vi "Parallel Loops - Pre izmene.vi"() -> ()   [LabVIEW 2016]
panel:
  out "Iter Akvizicija":i32
  out "Real":dbl
  out "Z":bool
  out "Y":bool
  out "X":bool
  in  "Treshold":dbl=1.0999999999999999 min=0.0 max=5.0 step=0.1
  out "Akvizicija":bool
  out "ACC1 Z":dbl
  out "ACC1 Y":dbl
  out "ACC1 X":dbl
  out "data":dynamicdata(graph)
  in  "Akvizicija - Error":string="N/A"
  out "Iter Sekvenca":i32
  in  "stop":bool
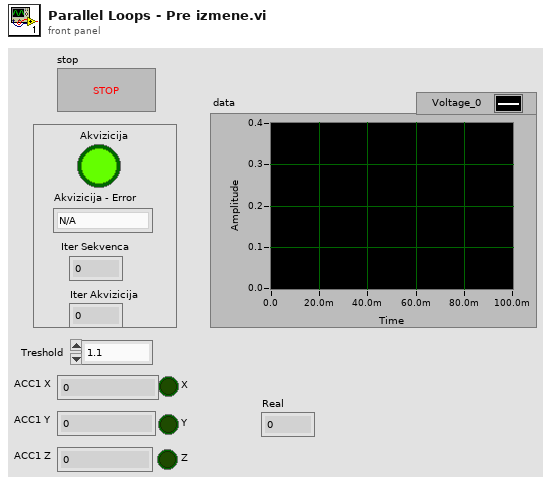
[diagram p1: front panel]
types:
  T1 = enum16{"open", "replace", "create", "open or create", "replace or create", "replace or create with confirmation"}
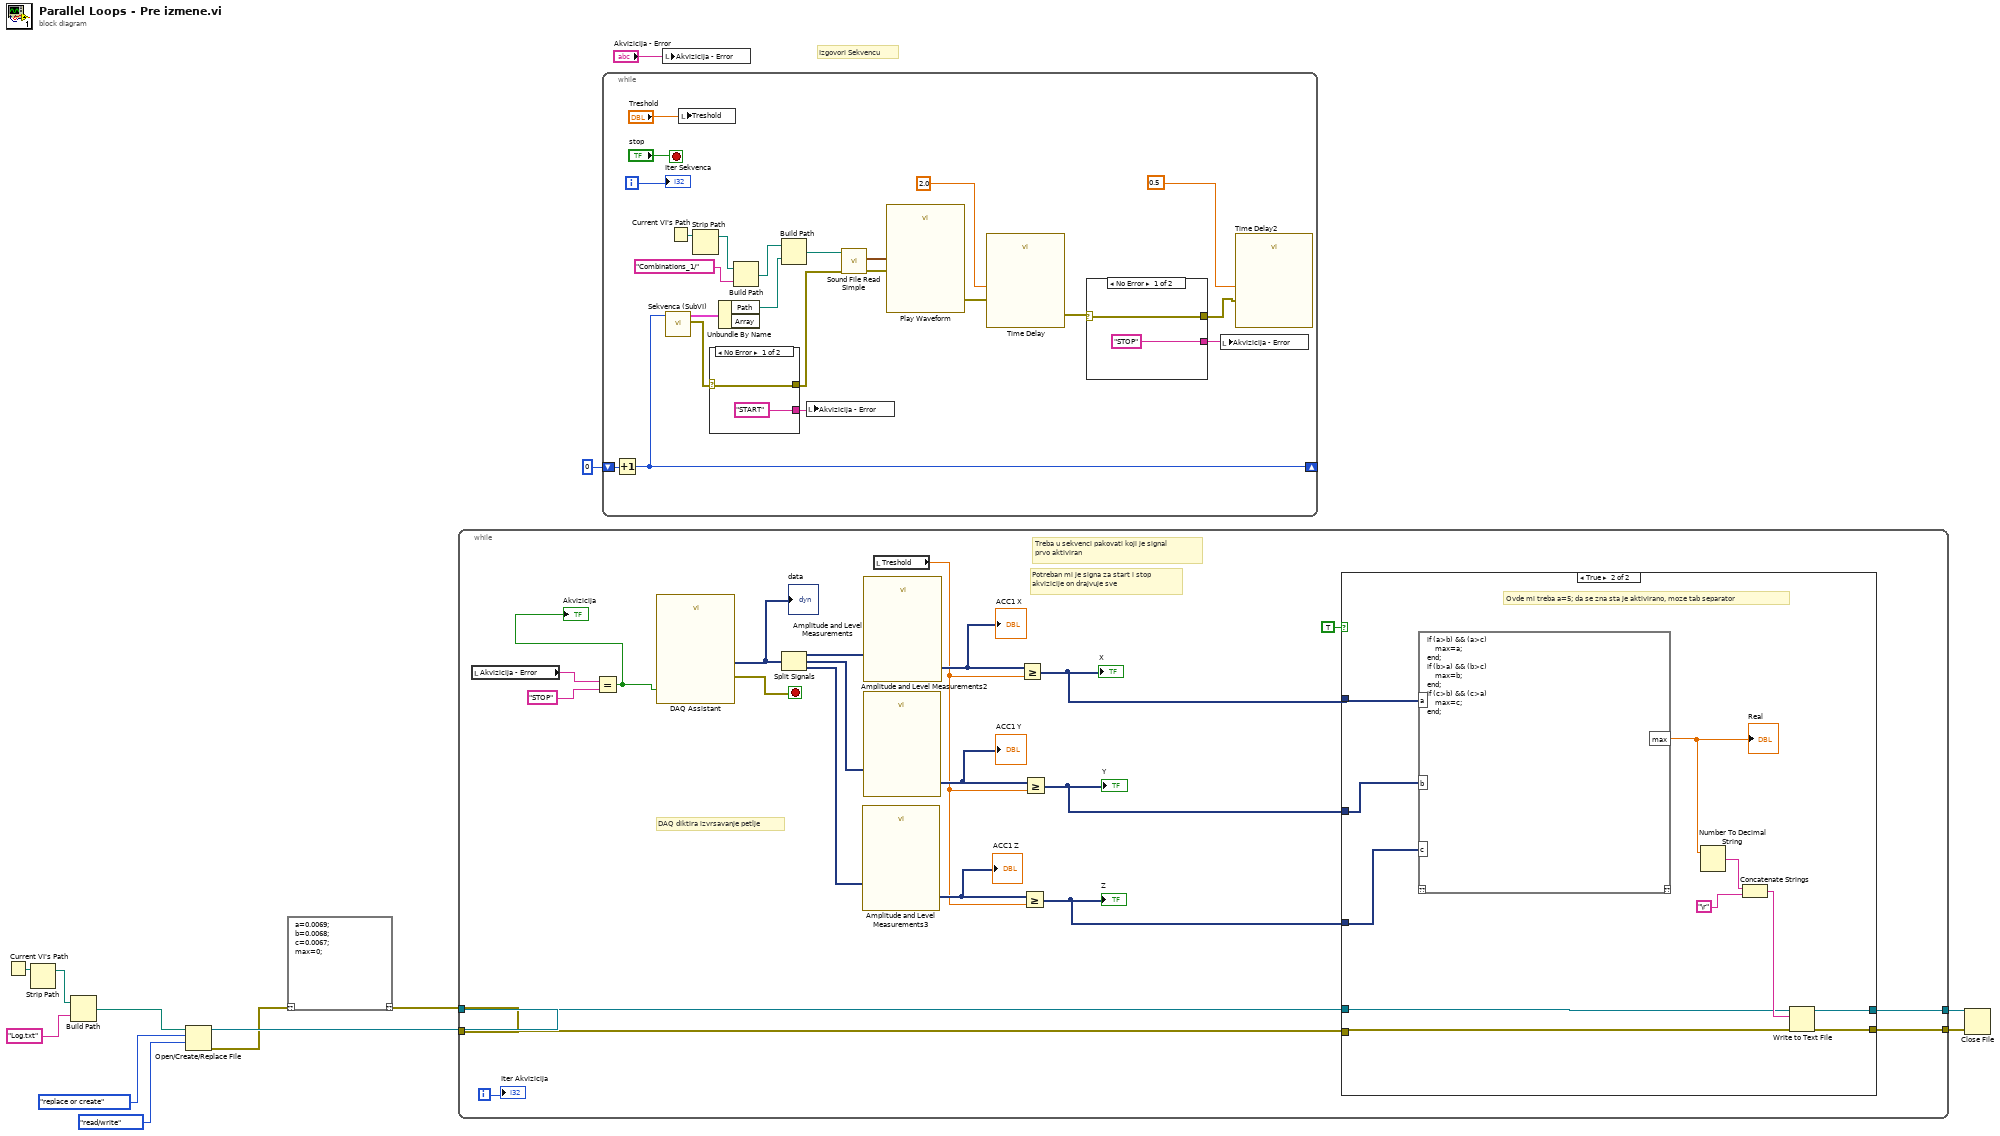
[diagram p0: block diagram]
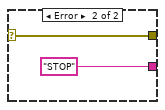
[diagram p3: hidden frame]
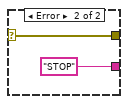
[diagram p4: hidden frame]
diagram:
  # "Izgovori Sekvencu"
  n1 = Current VI's Path() -> (path=w11:path)
  n2 = Strip Path(path=w11) -> (stripped path=w10:path)  [unwired: 1 out]
  n3 = Build Path(base path=w10, name or relative path="Log.txt") -> (appended path=w5:path)
  n4 = Open/Create/Replace File(file path (use dialog)=w5, operation (0:open)=T1."replace or create", access (0:read/write)=enum16{"read/write", "read-only", "write-only"}."read/write") -> (refnum out=w4:refnum<file>, error out=w3:errorcluster)  [unwired: 3 in, 1 out]
  n5 = script code="a=0.0069;\nb=0.0068;\nc=0.0067;\nmax=0;"("??"=w3) -> ("??"=w1:errorcluster)
  n6 = while {
    tunnel: w4 -> [w20]
    tunnel: [w19] -> w8
    tunnel: [w18] -> w7
    tunnel: w1 -> [w17]
    i -> [w14]
    stop <- w28 stop-if-true
    # "DAQ diktira izvrsavanje petlje"
    # "Potreban mi je signa za start i stop \nakvizicije on drajvuje sve"
    # "Treba u sekvenci pakovati koji je signal\nprvo aktiviran"
    n7 = local read "Akvizicija - Error"() -> (w29:string)
    n8 = Equal?(x=w29, y="STOP") -> (x = y?=w15:bool)
    "Akvizicija" <- w15
    n9 = call "DAQ Assistant"("stop (F)"=w15) -> ("data"=w31:dynamicdata, "error out"=w28:errorcluster)  [unwired: 15 in, 2 out]
    "data" <- w31
    n10 = Split Signals(w31) -> (w32:dynamicdata, w33:dynamicdata, w34:dynamicdata)  [unwired: 3 in]
    n11 = call "Amplitude and Level Measurements3"("Signals"=w34) -> ("Peak to Peak"=w25:dynamicdata)  [unwired: 13 in, 1 out]
    "ACC1 Z" <- w25
    n12 = call "Amplitude and Level Measurements2"("Signals"=w33) -> ("Peak to Peak"=w26:dynamicdata)  [unwired: 13 in, 1 out]
    "ACC1 Y" <- w26
    n13 = call "Amplitude and Level Measurements"("Signals"=w32) -> ("Peak to Peak"=w27:dynamicdata)  [unwired: 13 in, 1 out]
    "ACC1 X" <- w27
    n14 = local read "Treshold"() -> (w24:dbl)
    n15 = Greater Or Equal?(x=w27, y=w24) -> (x >= y?=w23:dynamicdata)
    "X" <- w23
    n16 = Greater Or Equal?(x=w25, y=w24) -> (x >= y?=w21:dynamicdata)
    "Z" <- w21
    n17 = Greater Or Equal?(x=w26, y=w24) -> (x >= y?=w22:dynamicdata)
    "Y" <- w22
    n18 = case shown="True" TRUE {
      tunnel: w23 -> [_ w47]
      tunnel: w22 -> [_ w46]
      tunnel: w21 -> [_ w45]
      tunnel: w20 -> [w35 w39]
      tunnel: [w35 w41] -> w19
      tunnel: [w36 w40] -> w18
      tunnel: w17 -> [w36 w37]
      frame False {
      }
      frame True {
        # "Ovde mi treba a=5; da se zna sta je aktivirano, moze tab separator"
        n19 = script code="if (a>b) && (a>c)\n    max=a; \nend;\nif (b>a) && (b>c)\n    max=b; \nend;\nif (c>b) && (c>a)\n    max=c; \nend;"("a"=w47, "b"=w46, "c"=w45) -> ("max"=w44:dbl)  [unwired: 1 in, 1 out]
        "Real" <- w44
        n20 = Number To Decimal String(number=w44) -> (decimal integer string=w43:string)  [unwired: 1 in]
        n21 = Concatenate Strings(w43, "\r") -> (w42:string)
        n22 = Write to Text File(file (use dialog)=w39, text=w42, error in=w37) -> (refnum out=w41:refnum<file>, error out=w40:errorcluster)  [unwired: 1 in, 1 out]
      }
    }
    "Iter Akvizicija" <- w14
  }
  n23 = while {
    shift-right: [w59] -> _
    shift-left: 0 -> [w60]
    i -> [w58]
    stop <- "stop" stop-if-true
    n24 = Increment(x=w60) -> (x+1=w59:i32)
    n25 = call "Sekvenca (SubVI).vi"("Ulaz"=w59) -> ("error out"=w57:errorcluster, "Cluster 41"=w62:cluster{"Path":path, "Array":dbl[]})  [unwired: 9 in]
    n26 = Current VI's Path() -> (path=w69:path)
    n27 = local write "Treshold"("Treshold") -> ()
    n28 = Strip Path(path=w69) -> (stripped path=w66:path)  [unwired: 1 out]
    n29 = case shown="No Error" w57 {
      selector: w57 -> [w75 w77]
      tunnel: ["START" "STOP"] -> w55
      tunnel: [w75 w77] -> w56
      frame No Error {
      }
      frame Error {
      }
    }
    n30 = Unbundle By Name(w62) -> ("Path"=w63:path)  [unwired: 1 out]
    n31 = Build Path(base path=w66, name or relative path="Combinations_1/") -> (appended path=w68:path)
    n32 = Build Path(base path=w68, name or relative path=w63) -> (appended path=w67:path)
    n33 = local write "Akvizicija - Error"(w55) -> ()
    n34 = call <vilib>:"Sound File Read Simple.vi"("error in (no error)"=w56, "path"=w67) -> ("error out"=w70:errorcluster, "data"=w64:waveform(dbl)[])  [unwired: 6 in, 2 out]
    n35 = call "Play Waveform"("Data"=w64, "error in"=w70) -> ("error out"=w53:errorcluster)  [unwired: 17 in]
    n36 = call "Time Delay"("error in (no error)"=w53, "Delay Time (s)"=2.0) -> ("error out"=w52:errorcluster)  [unwired: 9 in]
    n37 = case shown="No Error" w52 {
      selector: w52 -> [w71 w73]
      tunnel: ["STOP" "STOP"] -> w54
      tunnel: [w71 w73] -> w51
      frame No Error {
      }
      frame Error {
      }
    }
    n38 = local write "Akvizicija - Error"(w54) -> ()
    n39 = call "Time Delay2"("error in (no error)"=w51, "Delay Time (s)"=0.5) -> ()  [unwired: 9 in, 1 out]
    "Iter Sekvenca" <- w58
  }
  n40 = local write "Akvizicija - Error"("Akvizicija - Error") -> ()
  n41 = Close File(refnum=w8, error in=w7) -> ()  [unwired: 2 out]
